vi "cal_sub_bool_const_pos.vi"(0 "Disable String":string="OFF", 5 "1st sub node x position":i32, 7 "Last Control Position":cluster{"Left":i32, "Top":i32}, 9 "Last Function Position":cluster{"Left":i32, "Top":i32}, 11 "error in":errorcluster) -> (6 "Enable String Position":cluster{"Left":i32, "Top":i32}, 10 "Disable String Position":cluster{"Left":i32, "Top":i32}, 15 "error out":errorcluster)   [LabVIEW 2018]
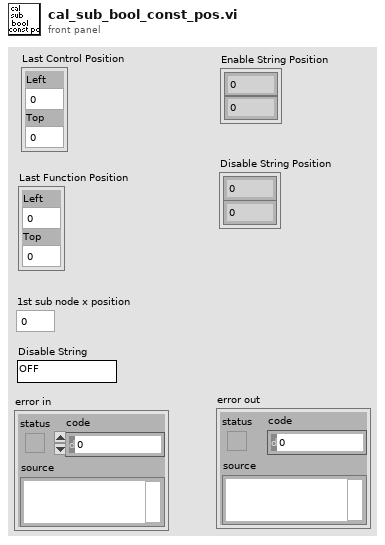
[diagram p1: front panel]
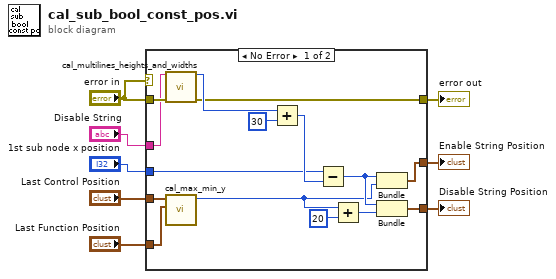
[diagram p0: block diagram]
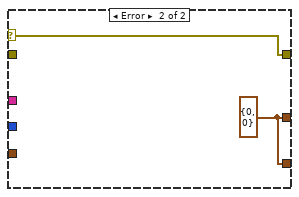
[diagram p2: hidden frame]
diagram:
  n1 = case shown="No Error" "error in" {
    selector: "error in" -> [_ w25]
    tunnel: [w19 w25] -> w8
    tunnel: "error in" -> [w18 _]
    tunnel: [w17 w24] -> w7
    tunnel: [w14 w24] -> w6
    tunnel: "Disable String" -> [w13 _]
    tunnel: "Last Control Position" -> [w12 _]
    tunnel: "Last Function Position" -> [w11 _]
    tunnel: "1st sub node x position" -> [w9 _]
    frame No Error {
      n2 = call "cal_multilines_heights_and_widths.vi"("Ring Command"=w13, "error in (no error)"=w18) -> ("BD Width"=w20:i32, "error out"=w19:errorcluster)  [unwired: 4 in, 8 out]
      n3 = call "cal_max_min_y.vi"("Position 2"=w11, "Position 1"=w12) -> ("max y"=w10:i32)  [unwired: 9 out]
      n4 = Add(x=w20, y=30) -> (x+y=w22:i32)
      n5 = Subtract(x=w9, y=w22) -> (x-y=w23:i32)
      n6 = Add(x=w10, y=20) -> (x+y=w15:i32)
      n7 = Bundle(w23, "max y"=w10) -> (w17:cluster{i32, "max y":i32})  [unwired: 1 out]
      n8 = Bundle(w23, w15) -> (w14:cluster{i32, i32})  [unwired: 1 out]
    }
    frame Error {
      w24 = cluster{i32, i32} {0, 0}
    }
  }
  "error out" <- w8
  "Enable String Position" <- w7
  "Disable String Position" <- w6
